vi "cDAQ Wait Digitize.vi"(8 "error in":errorcluster, 11 "cdaq session in":T3={"mclk [Hz]"=12800000.0, "ADC task"="", "mclk reference"="", "fs [Hz]"=50000.0, "queue adc cmd"=refnum, "queue adc data"=refnum, "adc proc ref"=refnum, "channels"=[], "last channels"=[], "timeout"=timestamp(0 s since 1904-01-01), "N"=1000} {"last channels"."Channel id" min=0 step=1; "channels"."Channel id" min=0 step=1}) -> (0 "error out":errorcluster, 1 "aux data":T2, 2 "sample data":T1, 3 "cdaq session out":T3={"mclk [Hz]"=12800000.0, "ADC task"="", "mclk reference"="", "fs [Hz]"=50000.0, "queue adc cmd"=refnum, "queue adc data"=refnum, "adc proc ref"=refnum, "channels"=[], "last channels"=[], "timeout"=timestamp(0 s since 1904-01-01), "N"=1000} {"last channels"."Channel id" min=0 step=1; "channels"."Channel id" min=0 step=1}, 5 "fetching done?":bool)   [LabVIEW 2013]
uses:
  cDAQ Session.ctl
  low_level_old/cdaq_anal_adc_command.ctl
  low_level_old/cdaq_anal_adc_data.ctl
  cDAQ Virtual Channel.ctl
  cDAQ Record Aux Data.ctl
  cDAQ Record Sample Data.ctl
  <vilib>/Utility/error.llb/Error Cluster From Error Code.vi
  <vilib>/ErrorRing/Error Ring.xnode
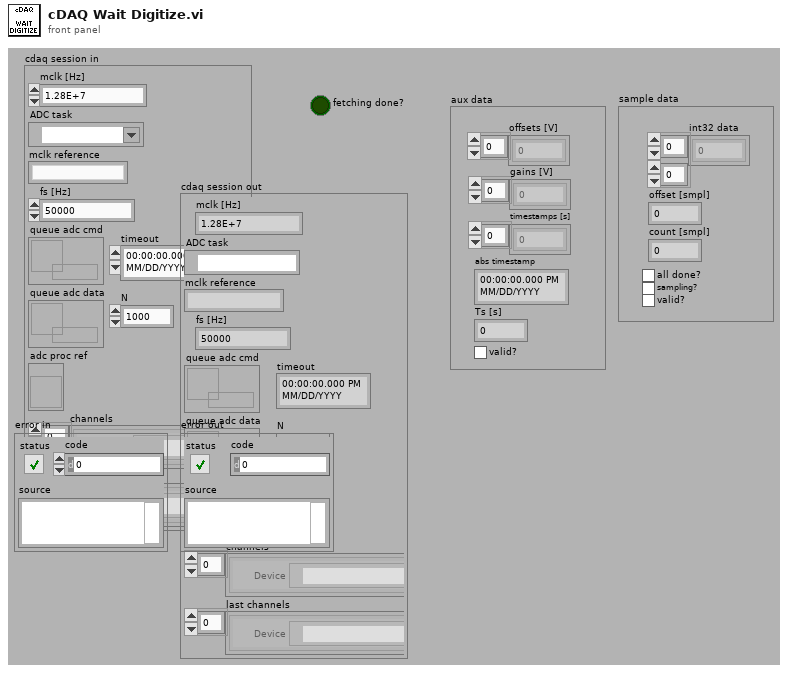
[diagram p1: front panel]
types:
  T1 = typedef "cDAQ Record Sample Data.ctl" = cluster{"int32 data":i32[][], "offset [smpl]":i64, "count [smpl]":i64, "all done?":bool, "sampling?":bool, "valid?":bool}
  T2 = typedef "cDAQ Record Aux Data.ctl" = cluster{"offsets [V]":dbl[], "gains [V]":dbl[], "timestamps [s]":dbl[], "abs timestamp":timestamp, "Ts [s]":dbl, "valid?":bool}
  T3 = typedef "cDAQ Session.ctl" = cluster{"mclk [Hz]":dbl, "ADC task":refnum<k21>, "mclk reference":string, "fs [Hz]":dbl, "queue adc cmd":refnum<queue>, "queue adc data":refnum<queue>, "adc proc ref":refnum<vi>, "channels":T4[], "last channels":T4[], "timeout":timestamp, "N":i32}
  T4 = typedef "cDAQ Virtual Channel.ctl" = cluster{"Device":tag, "Channel id":i32, "btn clr":bool, "btn up":bool, "btn down":bool}
  T5 = typedef "cdaq_anal_adc_data.ctl" = cluster{"wave":dbl[][], "timestamp [s]":dbl, "abs timestamp":timestamp, "Aborted":bool}
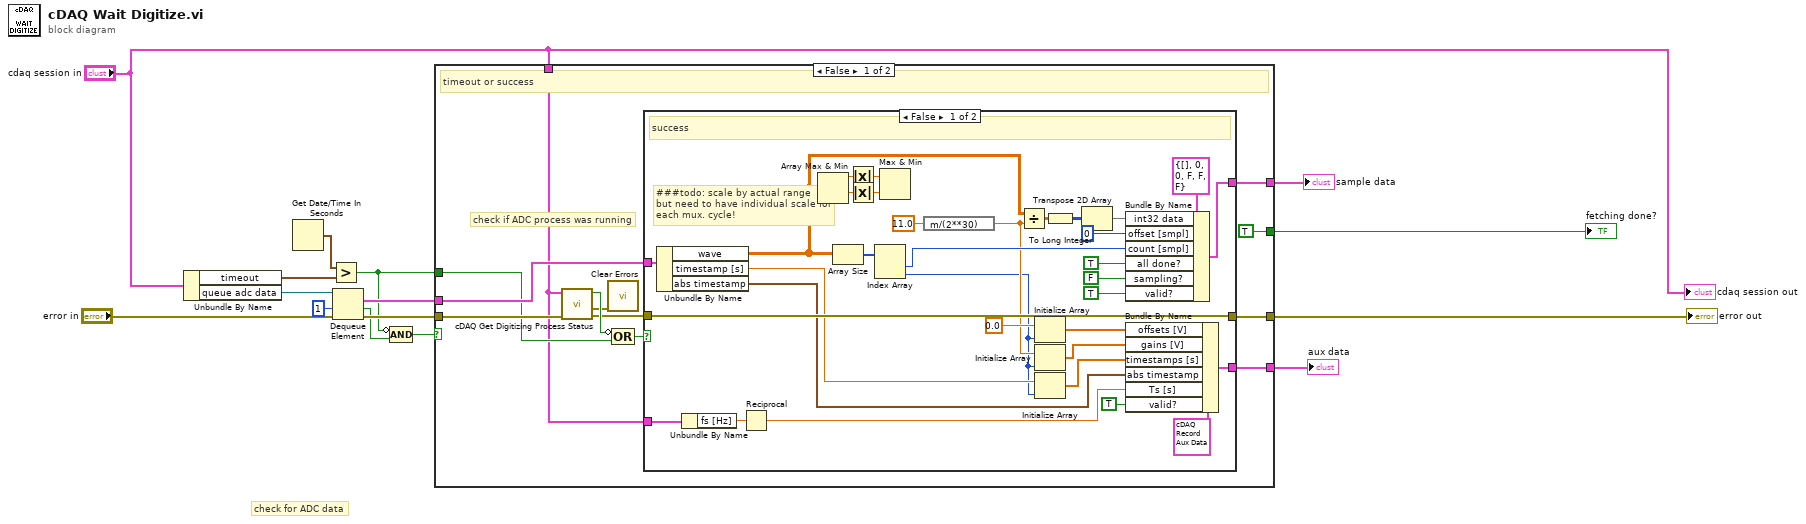
[diagram p0: block diagram]
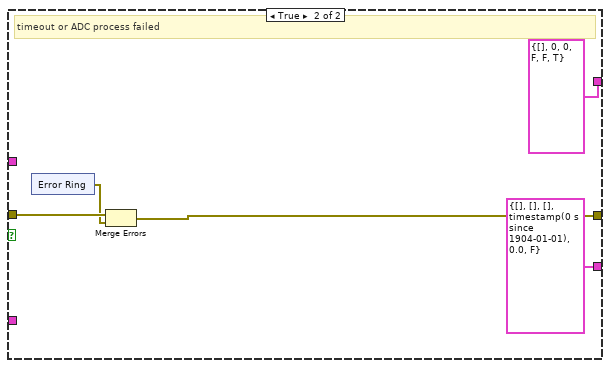
[diagram p2: hidden frame]
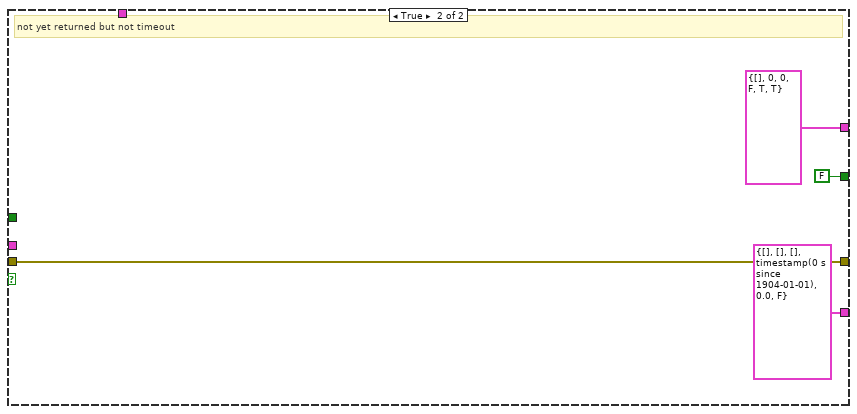
[diagram p3: hidden frame]
diagram:
  # "check for ADC data"
  n1 = Unbundle By Name("cdaq session in") -> ("timeout"=w7:timestamp, "queue adc data"=w11:refnum<queue>)
  n2 = Get Date/Time In Seconds() -> (seconds since 1Jan1904=w8:timestamp)
  n3 = Greater?(x=w8, y=w7) -> (0:w4:bool)
  n4 = Dequeue Element(queue=w11, timeout in ms (-1)=1, error in (no error)="error in") -> (element=w13:T5, timed out?=w5:bool, error out=w15:errorcluster)  [unwired: 1 out]
  n5 = Compound Arithmetic op=AND(invert w4, w5) -> (w6:bool)
  n6 = case shown="False" w6 {
    tunnel: w15 -> [w27 w74]
    tunnel: [w22 w74] -> w14
    tunnel: w13 -> [w21 _]
    tunnel: "cdaq session in" -> [w17 _]
    tunnel: w4 -> [w20 _]
    tunnel: [TRUE FALSE] -> w3
    tunnel: [w18 T1 {"int32 data"=[], "offset [smpl]"=0, "count [smpl]"=0, "all done?"=FALSE, "sampling?"=TRUE, "valid?"=TRUE} ("sample data")] -> w2
    tunnel: [w16 T2 {"offsets [V]"=[], "gains [V]"=[], "timestamps [s]"=[], "abs timestamp"=timestamp(0 s since 1904-01-01), "Ts [s]"=0.0, "valid?"=FALSE} ("aux data")] -> w1
    frame False {
      # "check if ADC process was running"
      # "timeout or success"
      n7 = call "cDAQ Get Digitizing Process Status.vi"("error in"=w27, "cdaq session"=w17) -> ("error out"=w24:errorcluster, "sweep error out"=w23:errorcluster, "is running"=w26:bool)  [unwired: 7 in]
      n8 = call <vilib>:"Clear Errors.vi"("error in (no error)"=w23) -> ()  [unwired: 6 in, 1 out]
      n9 = Compound Arithmetic op=OR(invert w26, w20) -> (w25:bool)
      n10 = case shown="False" w25 {
        tunnel: w24 -> [w60 w65]
        tunnel: [w60 w63] -> w22
        tunnel: w21 -> [w59 _]
        tunnel: [w46 T1 {"int32 data"=[], "offset [smpl]"=0, "count [smpl]"=0, "all done?"=FALSE, "sampling?"=FALSE, "valid?"=TRUE} ("sample data")] -> w18
        tunnel: w17 -> [w37 _]
        tunnel: [w32 T2 {"offsets [V]"=[], "gains [V]"=[], "timestamps [s]"=[], "abs timestamp"=timestamp(0 s since 1904-01-01), "Ts [s]"=0.0, "valid?"=FALSE} ("aux data")] -> w16
        frame False {
          # "###todo: scale by actual range\nbut need to have individual scale for \neach mux. cycle!"
          # "success"
          n11 = Unbundle By Name(w59) -> ("wave"=w30:dbl[][], "timestamp [s]"=w39:dbl, "abs timestamp"=w34:timestamp)
          n12 = Unbundle By Name(w37) -> ("fs [Hz]"=w36:dbl)
          n13 = Reciprocal(x=w36) -> (1/x=w35:dbl)
          n14 = Array Max & Min(array=w30) -> (max value=w56:dbl, min value=w57:dbl)  [unwired: 2 out]
          n15 = Array Size(array=w30) -> (size(s)=w51:i32[])
          n16 = Absolute Value(x=w56) -> (abs(x)=w54:dbl)
          n17 = Absolute Value(x=w57) -> (abs(x)=w55:dbl)
          n18 = Index Array(array=w51) -> (element #1=w50:i32, element #2=w38:i32)  [unwired: 2 in]
          n19 = Max & Min(x=w54, y=w55) -> ()  [unwired: 2 out]
          n20 = expression code="m/(2**30)"(11.0) -> (w41:dbl)
          n21 = Divide(x=w30, y=w41) -> (x/y=w53:dbl[][])
          n22 = Initialize Array(0.0, w38) -> (w44:dbl[])
          n23 = Initialize Array(w41, w38) -> (w42:dbl[])
          n24 = Initialize Array(w39, w38) -> (w40:dbl[])
          n25 = To Long Integer(number=w53) -> (32bit integer=w31:i32[][])
          n26 = Transpose 2D Array(2D array=w31) -> (transposed array=w29:i32[][])
          n27 = Bundle By Name(cluster=T1 {"int32 data"=[], "offset [smpl]"=0, "count [smpl]"=0, "all done?"=FALSE, "sampling?"=FALSE, "valid?"=FALSE} ("sample data"), "int32 data"=w29, "offset [smpl]"=i64 0, "count [smpl]"=w50, "all done?"=TRUE, "sampling?"=FALSE, "valid?"=TRUE) -> (w46:T1)
          n28 = Bundle By Name(cluster=T2 {"offsets [V]"=[], "gains [V]"=[], "timestamps [s]"=[], "abs timestamp"=timestamp(0 s since 1904-01-01), "Ts [s]"=0.0, "valid?"=FALSE} ("aux data"), "offsets [V]"=w44, "gains [V]"=w42, "timestamps [s]"=w40, "abs timestamp"=w34, "Ts [s]"=w35, "valid?"=TRUE) -> (w32:T2)
        }
        frame True {
          # "timeout or ADC process failed"
          n29 = xnode "Error Ring"() -> ("error out"=w64:errorcluster)
          n30 = Merge Errors(w65, w64) -> (w63:errorcluster)
        }
      }
    }
    frame True {
      # "not yet returned but not timeout"
    }
  }
  "error out" <- w14
  "fetching done?" <- w3
  "aux data" <- w1
  "sample data" <- w2
  "cdaq session out" <- "cdaq session in"
